vi "Update Inventario.vi"(8 "error in (no error)":errorcluster, 9 "Inventario":dbl, 10 "Index":i32, 11 "Soda_Actor in":refnum<class "Soda_Actor.lvclass">) -> (0 "error out":errorcluster, 3 "Soda_Actor out":refnum<class "Soda_Actor.lvclass">)   [LabVIEW 2019, in "Soda_Actor.lvlib" / "Soda_Actor.lvclass"]
uses:
  Soda_Actor.lvclass
  Soda_Actor.lvclass/Soda_Actor.ctl
  <vilib>/Utility/config.llb/Write Key (String).vi
  <vilib>/Utility/config.llb/NI_LVConfig.lvlib
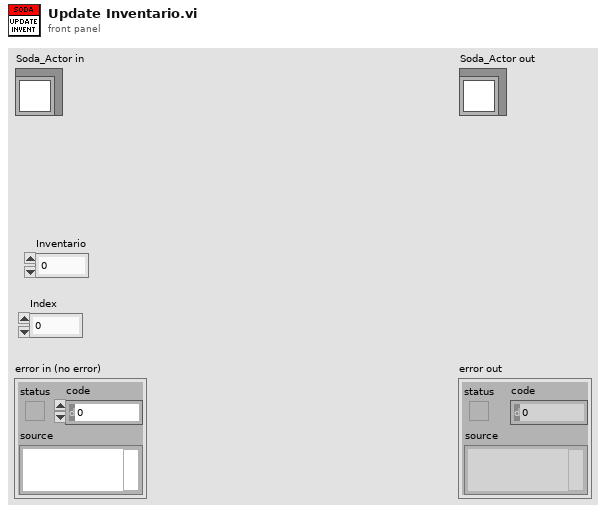
[diagram p1: front panel]
types:
  T1 = typedef "NI_LVConfig.lvlib/Config Data RefNum.ctl" = refnum<k1>
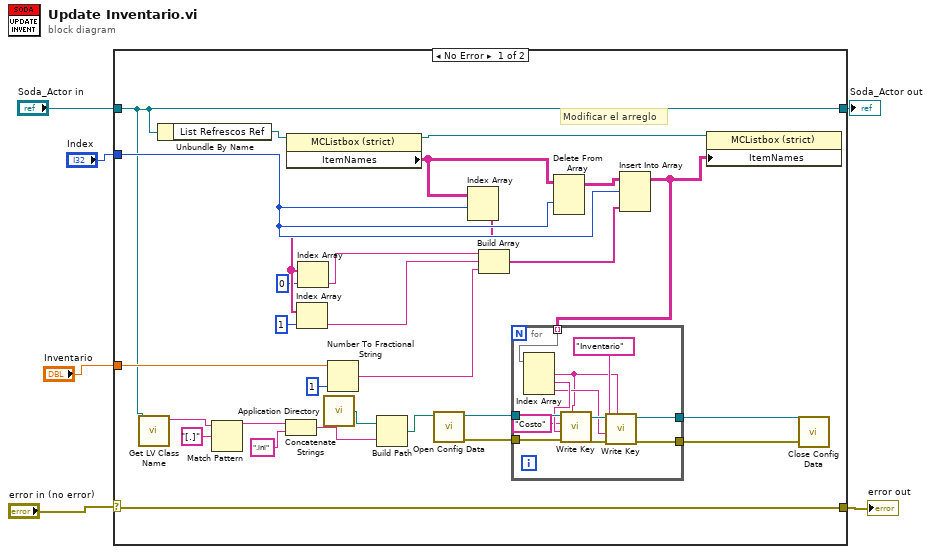
[diagram p0: block diagram]
diagram:
  n1 = case shown="No Error" "error in (no error)" {
    selector: "error in (no error)" -> [w34 w48]
    tunnel: [w34 w48] -> w5
    tunnel: [w13 w47] -> w3
    tunnel: "Soda_Actor in" -> [w13 w47]
    tunnel: "Index" -> [w15 _]
    tunnel: "Inventario" -> [w14 _]
    frame No Error {
      # "Modificar el arreglo"
      n2 = call <vilib>:"Get LV Class Name.vi"("object"=w13) -> ("class name"=w26:string)  [unwired: 9 in, 1 out]
      n3 = Unbundle By Name(w13) -> ("List Refrescos Ref"=w12:refnum<vi>)
      n4 = Match Pattern(string=w26, regular expression="[.]") -> (before substring=w25:string)  [unwired: 1 in, 3 out]
      n5 = Concatenate Strings(w25, ".ini" ("string")) -> (w22:string)
      n6 = property class="MCListbox (strict)"(reference=w12) -> (reference out=w32:refnum<vi>, "ItemNames"=w33:string[][])  [unwired: 1 in, 1 out]
      n7 = call <vilib>:"Application Directory.vi"() -> ("Application Directory"=w23:path)
      n8 = Number To Fractional String(number=w14, precision (6)=i16 1) -> (F-format string=w29:string)  [unwired: 2 in]
      n9 = Build Path(base path=w23, name or relative path=w22) -> (appended path=w21:path)
      n10 = call <vilib>:"Open Config Data.vi"("configuration file path"=w21) -> ("error out"=w19:errorcluster, "refnum"=w20:T1)  [unwired: 8 in, 1 out]
      n11 = Index Array(array=w33, index (row)=w15) -> (element=w11:string[])  [unwired: 1 in]
      n12 = Index Array(array=w11, index=1) -> (element=w7:string)
      n13 = Index Array(array=w11, index=0) -> (element=w8:string)
      n14 = Build Array(w8, w7, w29) -> (w28:string[])
      n15 = Delete From Array(array=w33, index (row)=w15) -> (array with subset deleted=w31:string[][])  [unwired: 2 in, 1 out]
      n16 = Insert Into Array(array=w31, index (row)=w15, new element=w28) -> (w18:string[][])  [unwired: 1 in]
      n17 = for {
        tunnel: w20 -> [w44]
        tunnel: w19 -> [w43]
        tunnel: w18 -> [w38] mode=indexing
        tunnel: [w36] -> w17
        tunnel: [w35] -> w16
        n18 = Index Array(array=w38) -> (element #1=w37:string, element #2=w42:string, element #3=w41:string)  [unwired: 3 in]
        n19 = call-poly <vilib>:"Write Key.vi"("section"=w37, "error in (no error)"=w43, "value"=w42, "key"="Costo", "refnum"=w44) -> ("error out"=w45:errorcluster, "refnum out"=w46:T1)  [unwired: 4 in, 1 out]
        n20 = call-poly <vilib>:"Write Key.vi"("section"=w37, "error in (no error)"=w45, "value"=w41, "key"="Inventario", "refnum"=w46) -> ("error out"=w36:errorcluster, "refnum out"=w35:T1)  [unwired: 4 in, 1 out]
      }
      n21 = property class="MCListbox (strict)"(reference=w32, "ItemNames"=w18) -> ()  [unwired: 1 in, 2 out]
      n22 = call <vilib>:"Close Config Data.vi"("error in (no error)"=w17, "refnum"=w16) -> ()  [unwired: 8 in, 2 out]
    }
    frame Error {
    }
  }
  "error out" <- w5
  "Soda_Actor out" <- w3
